vi "Kirigami_Measurement_WO_Filter_by_Hong-210412.vi"() -> ()   [LabVIEW 2015]
uses:
  <vilib>/Utility/file.llb/Write Delimited Spreadsheet (DBL).vi
panel:
  in  "Layer_type":string(combo) caption="L_type"
  in  "SA":string(combo) caption="S_amp(%)"
  in  "SR":string(combo) caption="S_Rate(mm/s)"
  in  "Suffix":string
  out "Dial_voltage":dbl(knob) caption="Voltage (V)" scale=-0.5..0.5 scale format="%#.3g"
  in  "Order":i8 caption="Order\nD : 3"
  out "Filtered voltage":dbl[](graph)
  out "Time (s)":dbl format="%#.2f"
  out "Time_count":dbl caption="Count_time (ms)" format="%#_6f"
  in  "Path_dir":path caption="Log file path (파일은 자동 생성. 디렉토리만 지정해주면 됨)\n되도록 엑세스가 빠른 디스크를 경로로 지정하세요."
  out "T_log_period":dbl caption="Data period (ms)\n>= 10 recommended."
  in  "B_STOP":bool caption="STOP"
  out "Count":u32 caption="Iter_count"
  in  "Str_ft":string(combo) caption="Film type"
  in  "Str_kl":string(combo) caption="Kirigami Layer"
  out "Result filename":string
  in  "B_logging":bool caption="Logging"
  in  "B_default":bool caption="Set to default"
  out "N_s":u16 caption="N of samples per log\n= (H/W s. r.)/(Logging rate)\nMUST be bigger than 10"
  in  "F_s_log":u16=1 caption="Data rate(Hz)\n<= 100 recommended\nD : 100 Hz" min=1 max=48000
  in  "F_s_hw":u16 caption="DAQ sampling rate(Hz)\nD : 10000 Hz"
  in  "F_h":dbl caption="Upper freq.\n(Bandpass/Bandstop ONLY)\nD : 60 Hz"
  in  "F_l":dbl caption="Lower freq.\nD : 30 Hz"
  out "F_s":dbl caption="Sampling rate\n(Hz)"
  out "Raw voltage":dbl[](graph)
  # "Kirigami sensor voltage measurement"
  # "- SeongHeon Hong, Apr 10th, 2021 \nIDIM internship student"
  # "┌-------┬-----┬-----┬-----┬------┐\n|    o          |        |        |        o    |\n|    o          |        |        |        o    |\n└-------┴-----┴-----┴-----┴------┘"
  # "- NI USB-6009\n- Connect (+) terminal to pin 3\n- Connect (-) terminal to pin 2"
  # "Apply Filter"
  # "DAQ settings"
  # "파일 출력하려면 Logging 버튼 On 하고, 빈칸 남겨두지 마세요."
  # "File I/O settings"
  # "Modification not required\nin most cases"
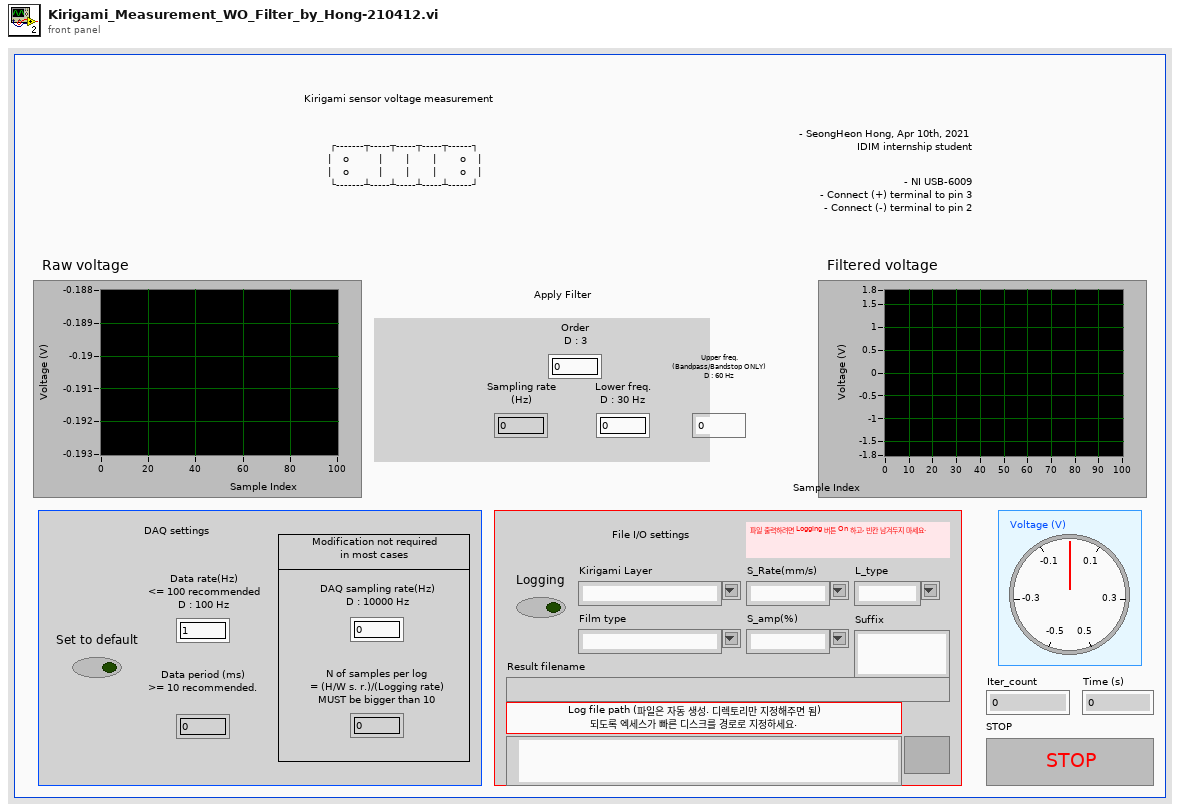
[diagram p1: front panel]
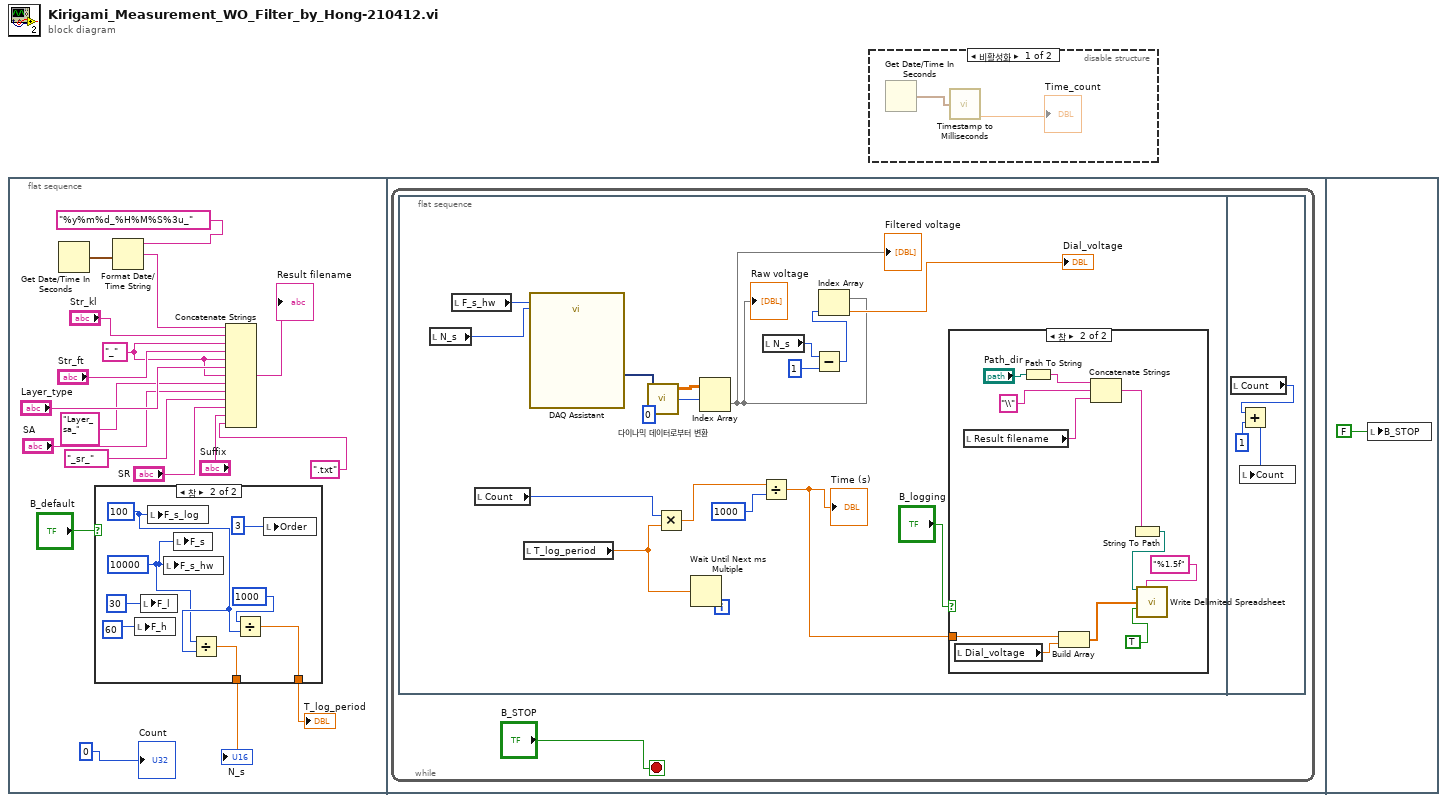
[diagram p0: block diagram]
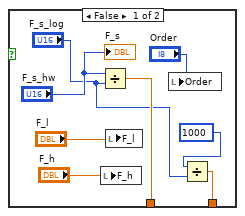
[diagram p3: hidden frame]
diagram:
  n1 = flat-sequence {
    frame #0 {
      w7 = "_"
      n2 = Get Date/Time In Seconds() -> (seconds since 1Jan1904=w14:timestamp)
      n3 = case shown="참" "B_default" {
        tunnel: [w22 w31] -> w11
        tunnel: [w21 w29] -> w10
        frame False {
          n4 = Divide(x="F_s_hw", y="F_s_log") -> (x/y=w21:dbl)
          n5 = local write "F_h"("F_h") -> ()
          n6 = local write "F_l"("F_l") -> ()
          n7 = local write "Order"("Order") -> ()
          n8 = Divide(x=1000, y="F_s_log") -> (x/y=w22:dbl)
          "F_s" <- "F_s_hw"
        }
        frame True {
          w27 = 10000
          w30 = 100
          n9 = local write "F_h"(60) -> ()
          n10 = local write "F_l"(30) -> ()
          n11 = local write "F_s_log"(w30) -> ()
          n12 = local write "F_s_hw"(w27) -> ()
          n13 = local write "F_s"(w27) -> ()
          n14 = Divide(x=w27, y=w30) -> (x/y=w29:dbl)
          n15 = Divide(x=1000, y=w30) -> (x/y=w31:dbl)
          n16 = local write "Order"(3) -> ()
        }
      }
      "T_log_period" <- w11
      "N_s" <- w10
      n17 = Format Date/Time String(time format string (%c)="%y%m%d_%H%M%S%3u_", seconds (now)=w14) -> (date/time string=w16:string)  [unwired: 1 in]
      n18 = Concatenate Strings(w16, "Str_kl", w7, "Str_ft", w7, "Layer_type", w7, "Layer_sa_", "SA", "_sr_", "SR", "Suffix", ".txt") -> (→"Result filename":string)
      "Count" <- 0
    }
    frame #1 {
      n19 = while {
        stop <- "B_STOP" stop-if-true
        n20 = flat-sequence {
          frame #0 {
            n21 = local read "N_s"() -> (w51:u16)
            n22 = local read "F_s_hw"() -> (w47:u16)
            n23 = local read "Count"() -> (w45:u32)
            n24 = local read "T_log_period"() -> (w44:dbl)
            n25 = call "DAQ Assistant"("속도"=w47, "샘플 개수"=w51) -> ("data"=w50:dynamicdata)  [unwired: 14 in, 3 out]
            n26 = call "다이나믹 데이터로부터 변환"("Dynamic Data Type"=w50) -> ("Array"=w48:dbl[][])  [unwired: 3 in]
            n27 = Multiply(x=w45, y=w44) -> (x*y=w42:dbl)
            n28 = Wait Until Next ms Multiple(millisecond multiple=w44) -> ()  [unwired: 1 out]
            n29 = Index Array(array=w48, index (row)=u32 0) -> (element=w36:dbl[])  [unwired: 1 in]
            "Raw voltage" <- w36
            "Filtered voltage" <- w36
            n30 = Divide(x=w42, y=1000) -> (x/y=w40:dbl)
            "Time (s)" <- w40
            n31 = local read "N_s"() -> (w38:u16)
            n32 = Subtract(x=w38, y=u32 1) -> (x-y=w37:u32)
            n33 = Index Array(array=w36, index=w37) -> (element=→"Dial_voltage":dbl)
            n34 = case shown="참" "B_logging" {
              tunnel: w40 -> [_ w53]
              frame False {
              }
              frame True {
                n35 = local read "Dial_voltage"() -> (w52:dbl)
                n36 = local read "Result filename"() -> (w55:string)
                n37 = Path To String(path="Path_dir") -> (string=w61:string)
                n38 = Build Array(w53, w52) -> (w57:dbl[])
                n39 = Concatenate Strings(w61, "\\", w55) -> (w60:string)
                n40 = String To Path(string=w60) -> (path=w59:path)
                n41 = call-poly <vilib>:"Write Delimited Spreadsheet.vi"("file path (dialog if empty)"=w59, "format (%.3f)"="%1.5f", "1D data"=w57, "append to file? (F)"=TRUE) -> ()  [unwired: 10 in, 2 out]
              }
            }
          }
          frame #1 {
            n42 = local read "Count"() -> (w65:u32)
            n43 = Add(x=w65, y=1) -> (x+y=w63:u32)
            n44 = local write "Count"(w63) -> ()
          }
        }
      }
    }
    frame #2 {
      n45 = local write "B_STOP"(FALSE) -> ()
    }
  }
  n46 = disable-structure shown="비활성화" {
    frame Disabled {
      n47 = Get Date/Time In Seconds() -> (seconds since 1Jan1904=w67:timestamp)
      n48 = call "Timestamp to Milliseconds.vi"("Timestamp In"=w67) -> ("Seconds"=→"Time_count":dbl)  [unwired: 4 in, 3 out]
    }
    frame Enabled {
    }
  }
